vi "Identities.vi"(8 "error in (no error)":errorcluster, 11 "AbortAPI in":refnum<class "AbortAPI.lvclass">) -> (0 "error out":errorcluster, 2 "Identities":refnum<class "Identity.lvclass">[](array[class]), 3 "AbortAPI out":refnum<class "AbortAPI.lvclass">)   [LabVIEW 2020, in "Volatus.lvlib" / "AbortAPI.lvclass"]
uses:
  AbortAPI.lvclass
  Identity/Identity.lvclass
  AbortIdentity/AbortIdentity.lvclass
  C:/dev/lv20CE/relink/lv-volatus/Volatus/Identity/Identity.lvclass
  AbortAPI.lvclass/AbortAPI.ctl
  C:/dev/lv20CE/relink/lv-volatus/Volatus/AbortIdentity/AbortIdentity.lvclass
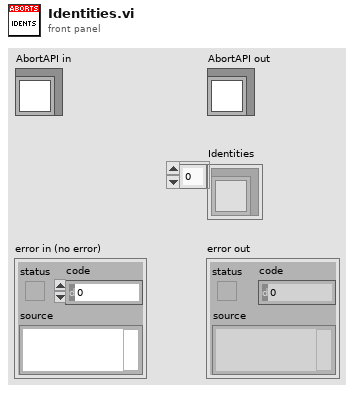
[diagram p1: front panel]
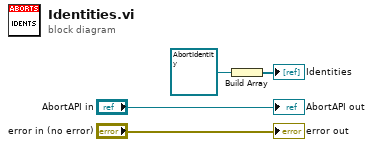
[diagram p0: block diagram]
diagram:
  n1 = Build Array(refnum<class "AbortIdentity.lvclass"> refnum ("Volatus:AbortIdentity.lvclass")) -> (→"Identities":refnum<class "AbortIdentity.lvclass">[])
  "error out" <- "error in (no error)"
  "AbortAPI out" <- "AbortAPI in"
